vi "Update Chart.vi"(8 "error in (no error)":errorcluster, 10 "Variant":variant, 11 "MultiSubscriber in":refnum<class "MultiSubscriber.lvclass">) -> (0 "error out":errorcluster, 3 "MultiSubscriber out":refnum<class "MultiSubscriber.lvclass">)   [LabVIEW 2015, in "TestViewables.lvlib" / "MultiSubscriber.lvclass"]
doc: "<License>\nCopyright © 2017 Composed Systems, LLC | All rights reserved\nwww.composed.io\n\nAuthor: Ethan Stern <ethan.stern@composed.io>\n\nThis software is provided \"AS IS\" WITHOUT WARRANTIES, either express or implied, AND IS FOR EDUCATIONAL PURPOSES ONLY.\n</License>"
uses:
  MultiSubscriber.lvclass
  Framework/IViewable/IViewable/IViewable.lvclass/IViewable.ctl
  MultiSubscriber.lvclass/MultiSubscriber.ctl
  Framework/IViewable/IViewable/IViewable.lvclass
panel:
  out "size(s)":i32
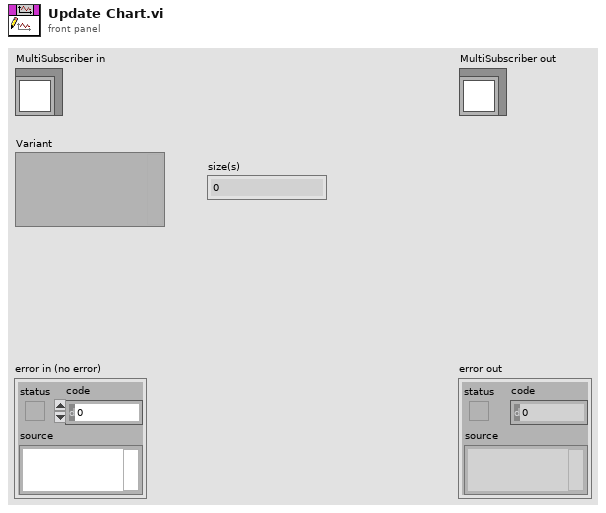
[diagram p1: front panel]
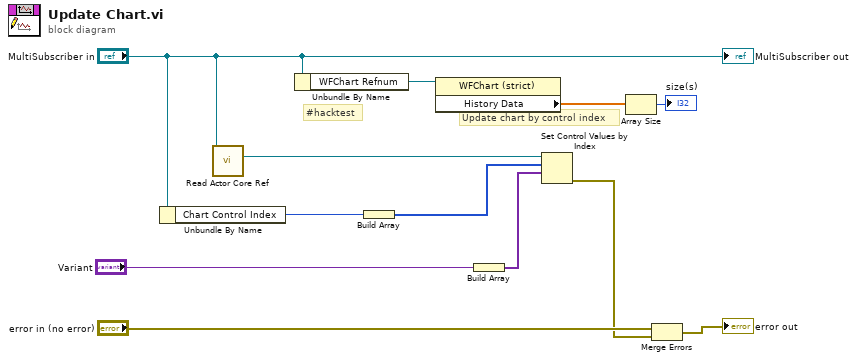
[diagram p0: block diagram]
diagram:
  # "#hacktest"
  # "Update chart by control index"
  n1 = Unbundle By Name("MultiSubscriber in") -> ("Chart Control Index"=w7:i32)
  n2 = call "Read Actor Core Ref.vi"("IViewable In"="MultiSubscriber in") -> ("Actor Core Ref"=w10:refnum<vi>)  [unwired: 8 in, 2 out]
  n3 = Unbundle By Name("MultiSubscriber in") -> ("WFChart Refnum"=w3:refnum<vi>)
  n4 = Build Array(w7) -> (w6:i32[])
  n5 = property class="WFChart (strict)"(reference=w3) -> ("History Data"=w2:dbl[])  [unwired: 1 in, 2 out]
  n6 = Build Array("Variant") -> (w8:variant[])
  n7 = Set Control Values by Index(0:w10, 1:w6, 2:w8) -> (11:w5:errorcluster)  [unwired: 1 in]
  n8 = Array Size(array=w2) -> (size(s)=→"size(s)":i32)
  n9 = Merge Errors("error in (no error)", w5) -> (→"error out":errorcluster)
  "MultiSubscriber out" <- "MultiSubscriber in"
